vi "Simple Drive Shifting COde.vi"   [LabVIEW 2012]
uses:
  <vilib>/Rock Robotics/WPI/DriverStation/DriverStationLCD/WPI_DriverStationLCDLCDLine.ctl
  Robot Global Data.vi
  <vilib>/Rock Robotics/WPI/Solenoid/Deprecated/WPI_SolenoidSetBool.vi
types:
  T1 = typedef "WPI_DriverStationLCDLCDLine.ctl" = enum16{"Main - Line 1", "User - Line 2", "User - Line 3", "User - Line 4", "User - Line 5", "User - Line 6"}
  T2 = typedef "WPI_SolenoidDevRef.ctl" = cluster{"DevStatus":errorcluster, "Solenoid Module":T3, "Forward Solenoid Channel":T4, "Reverse Solenoid Channel":T4}
  T3 = typedef "FPGA_TypedefSolenoidModule.ctl" = enum16{"Solenoid Module 1", "Solenoid Module 2"}
  T4 = typedef "WPI_SolenoidChannel.ctl" = enum8{"Solenoid 1", "Solenoid 2", "Solenoid 3", "Solenoid 4", "Solenoid 5", "Solenoid 6", "Solenoid 7", "Solenoid 8", "Invalid"}
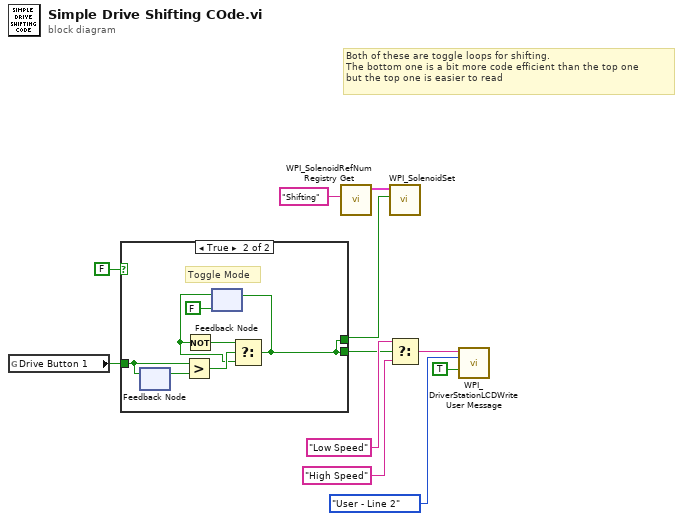
[diagram p0: block diagram]
diagram:
  # "Both of these are toggle loops for shifting.\nThe bottom one is a bit more code efficient than the top one\nbut the top one is easier to read"
  n1 = global read "Robot Global Data.vi" "Drive Button 1"() -> (w11:bool)
  n2 = case shown="True" FALSE {
    tunnel: w11 -> [w12 w19]
    tunnel: [w12 w13] -> w5
    tunnel: [w12 w13] -> w3
    frame False {
      # "Speed Burst Mode"
    }
    frame True {
      # "Toggle Mode"
      n3 = feedback #1() -> (w18:bool)  [unwired: 1 in]
      n4 = feedback-in #1(w19) -> ()
      n5 = Greater?(x=w19, y=w18) -> (0:w17:bool)
      n6 = feedback #2(FALSE) -> (w15:bool)
      n7 = Not(x=w15) -> (.not. x?=w16:bool)
      n8 = Select(t=w16, s=w17, f=w15) -> (s? t:f=w13:bool)
      n9 = feedback-in #2(w13) -> ()
    }
  }
  n10 = call <vilib>:"WPI_SolenoidRefNum Registry Get.vi"("refnum name"="Shifting") -> ("SolenoidDevRef"=w2:T2)  [unwired: 9 in, 1 out]
  n11 = call-poly <vilib>:"WPI_SolenoidSet.vi"("Value"=w3, "SolenoidDevRef"=w2) -> ()  [unwired: 8 in, 2 out]
  n12 = Select(t="Low Speed", s=w5, f="High Speed" ("line text")) -> (s? t:f=w7:string)
  n13 = call <vilib>:"WPI_DriverStationLCDWrite User Message.vi"("line text"=w7, "line"=WPI_DriverStationLCDLCDLine."User - Line 2", "clear line before write (T)"=TRUE) -> ()  [unwired: 12 in, 1 out]
